vi "Hardware In - NI 9862 (NOx).vi"() -> ()   [LabVIEW 2015, in "ECS-RT.lvlib"]
uses:
  ECS-RT.lvlib
  Globals/NOx Global.vi
panel:
  out "NOx1 Data":T1={"NOx (ppm)"=0, "O2 (%)"=0.0, "Sensor Supply Status"=3, "Sensor Temperature Status"=12, "NOx Signal Status"=48, "O2 Signal Status"=192, "Heater Mode Status"=96, "Heater Circuit Status"=31, "NOx Circuit Status"=31, "O2 Circuit Status"=31, "NOx Sensor Module Present"=FALSE} {"Heater Mode Status" items=["AUTO MODE"=0, "HEATUP SLOPE 3 OR 4"=32, "HEATUP SLOPE 1 OR 2"=64, "HEATER OFF / PREHEAT"=96]; "O2 Circuit Status" items=["OPEN WIRE"=3, "SHORT CIRCUIT"=5, "NO ERROR"=31]; "NOx Circuit Status" items=["OPEN WIRE"=3, "SHORT CIRCUIT"=5, "NO ERROR"=31]; "Heater Circuit Status" items=["OPEN WIRE"=3, "SHORT CIRCUIT"=5, "NO ERROR"=31]; "Sensor Temperature Status" items=["NOT AT TEMPERATURE"=0, "AT TEMPERATURE"=4, "ERROR"=8, "NOT AVAILABLE"=12]; "O2 Signal Status" items=["NOT VALID"=0, "VALID"=64, "ERROR"=128, "NOT AVAILABLE"=192]; "NOx Signal Status" items=["NOT VALID"=0, "VALID"=16, "ERROR"=32, "NOT AVAILABLE"=48]; "Sensor Supply Status" items=["NOT IN RANGE", "SUPPLY IN RANGE", "ERROR", "NOT AVAILABLE"]}
  out "NOx2 Data":T1={"NOx (ppm)"=0, "O2 (%)"=0.0, "Sensor Supply Status"=3, "Sensor Temperature Status"=12, "NOx Signal Status"=48, "O2 Signal Status"=192, "Heater Mode Status"=96, "Heater Circuit Status"=31, "NOx Circuit Status"=31, "O2 Circuit Status"=31, "NOx Sensor Module Present"=FALSE} {"Heater Mode Status" items=["AUTO MODE"=0, "HEATUP SLOPE 3 OR 4"=32, "HEATUP SLOPE 1 OR 2"=64, "HEATER OFF / PREHEAT"=96]; "O2 Circuit Status" items=["OPEN WIRE"=3, "SHORT CIRCUIT"=5, "NO ERROR"=31]; "NOx Circuit Status" items=["OPEN WIRE"=3, "SHORT CIRCUIT"=5, "NO ERROR"=31]; "Heater Circuit Status" items=["OPEN WIRE"=3, "SHORT CIRCUIT"=5, "NO ERROR"=31]; "Sensor Temperature Status" items=["NOT AT TEMPERATURE"=0, "AT TEMPERATURE"=4, "ERROR"=8, "NOT AVAILABLE"=12]; "O2 Signal Status" items=["NOT VALID"=0, "VALID"=64, "ERROR"=128, "NOT AVAILABLE"=192]; "NOx Signal Status" items=["NOT VALID"=0, "VALID"=16, "ERROR"=32, "NOT AVAILABLE"=48]; "Sensor Supply Status" items=["NOT IN RANGE", "SUPPLY IN RANGE", "ERROR", "NOT AVAILABLE"]}
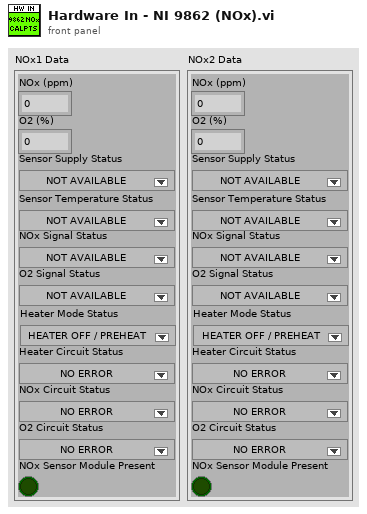
[diagram p1: front panel]
types:
  T1 = cluster{"NOx (ppm)":i16, "O2 (%)":sgl, "Sensor Supply Status":u8, "Sensor Temperature Status":u8, "NOx Signal Status":u8, "O2 Signal Status":u8, "Heater Mode Status":u8, "Heater Circuit Status":u8, "NOx Circuit Status":u8, "O2 Circuit Status":u8, "NOx Sensor Module Present":bool}
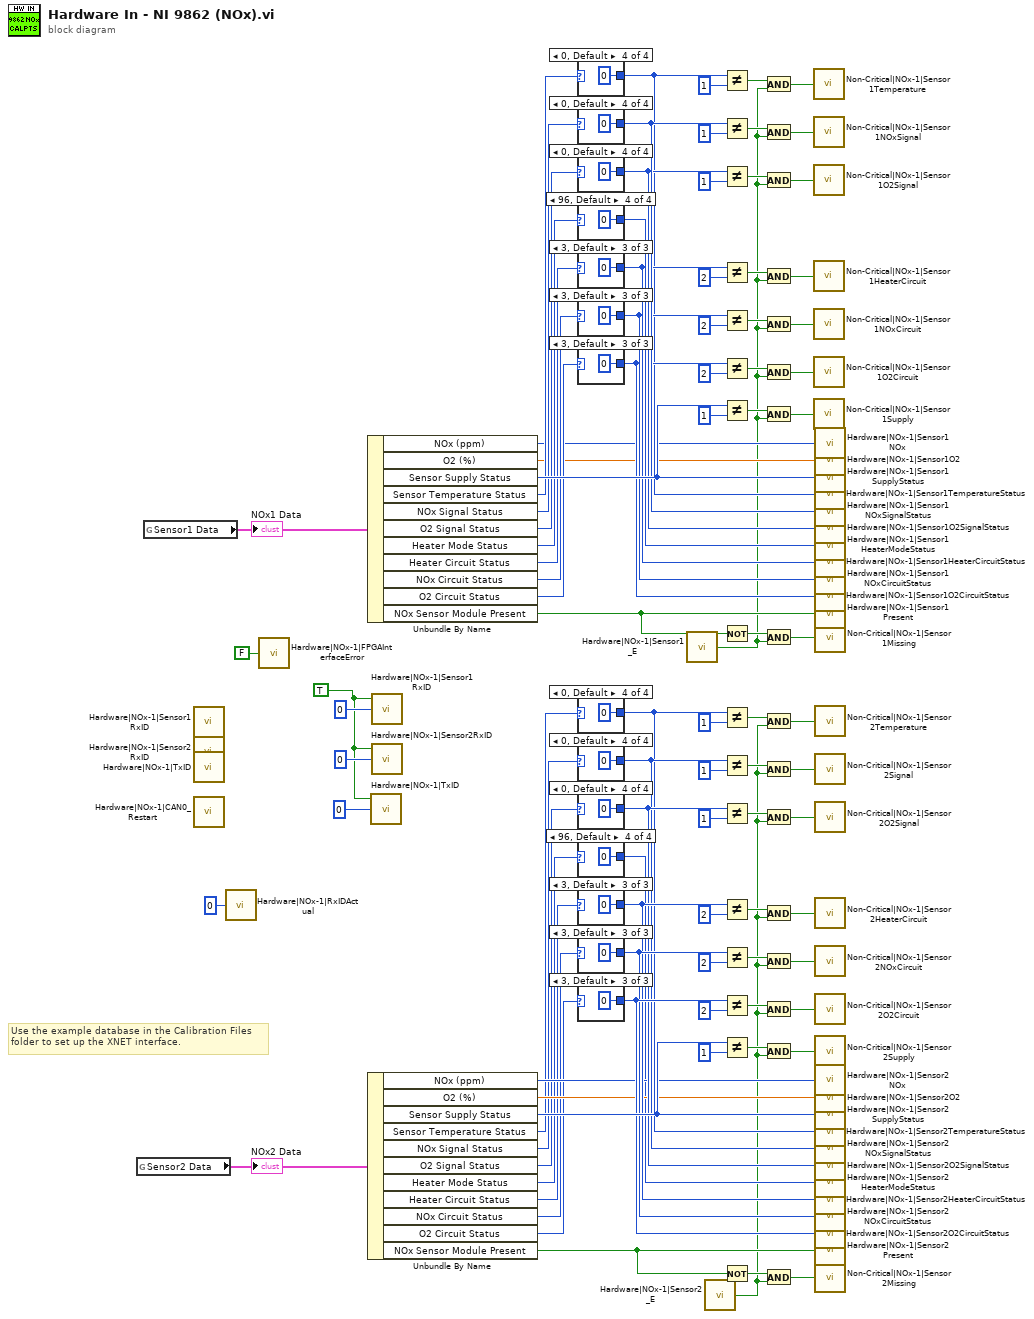
[diagram p0: block diagram]
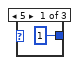
[diagram p2: hidden frame]
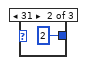
[diagram p3: hidden frame]
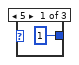
[diagram p4: hidden frame]
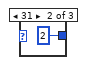
[diagram p5: hidden frame]
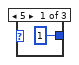
[diagram p6: hidden frame]
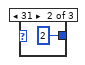
[diagram p7: hidden frame]
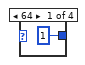
[diagram p8: hidden frame]
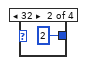
[diagram p9: hidden frame]
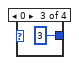
[diagram p10: hidden frame]
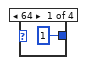
[diagram p11: hidden frame]
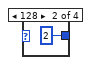
[diagram p12: hidden frame]
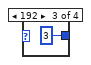
[diagram p13: hidden frame]
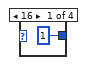
[diagram p14: hidden frame]
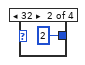
[diagram p15: hidden frame]
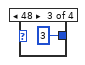
[diagram p16: hidden frame]
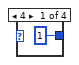
[diagram p17: hidden frame]
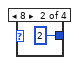
[diagram p18: hidden frame]
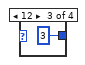
[diagram p19: hidden frame]
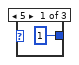
[diagram p20: hidden frame]
diagram:
  w3 = TRUE ("Adapt")
  # "Use the example database in the Calibration Files\nfolder to set up the XNET interface."
  n1 = global read "NOx Global.vi" "Sensor2 Data"() -> (w8:T1)
  "NOx2 Data" <- w8
  n2 = global read "NOx Global.vi" "Sensor1 Data"() -> (w7:T1)
  "NOx1 Data" <- w7
  n3 = call "Hardware|NOx-1|Sensor1RxID"() -> ()  [unwired: 1 out]
  n4 = call "Hardware|NOx-1|Sensor2RxID"() -> ()  [unwired: 1 out]
  n5 = call "Hardware|NOx-1|TxID"() -> ()  [unwired: 1 out]
  n6 = call "Hardware|NOx-1|CAN0_Restart"() -> ()  [unwired: 1 out]
  n7 = call "Hardware|NOx-1|RxIDActual"("Value"=u32 0) -> ()
  n8 = call "Hardware|NOx-1|FPGAInterfaceError"("Value"=FALSE) -> ()
  n9 = Unbundle By Name(w7) -> ("NOx (ppm)"=w43:i16, "O2 (%)"=w44:sgl, "Sensor Supply Status"=w76:u8, "Sensor Temperature Status"=w45:u8, "NOx Signal Status"=w46:u8, "O2 Signal Status"=w47:u8, "Heater Mode Status"=w48:u8, "Heater Circuit Status"=w49:u8, "NOx Circuit Status"=w50:u8, "O2 Circuit Status"=w51:u8, "NOx Sensor Module Present"=w77:bool)
  n10 = Unbundle By Name(w8) -> ("NOx (ppm)"=w61:i16, "O2 (%)"=w60:sgl, "Sensor Supply Status"=w91:u8, "Sensor Temperature Status"=w59:u8, "NOx Signal Status"=w58:u8, "O2 Signal Status"=w57:u8, "Heater Mode Status"=w55:u8, "Heater Circuit Status"=w54:u8, "NOx Circuit Status"=w53:u8, "O2 Circuit Status"=w52:u8, "NOx Sensor Module Present"=w92:bool)
  n11 = call "Hardware|NOx-1|TxID"("Value"=u32 0, "Adapt"=w3) -> ()  [unwired: 1 in]
  n12 = call "Hardware|NOx-1|Sensor1RxID"("Value"=u32 0, "Adapt"=w3) -> ()  [unwired: 1 in]
  n13 = call "Hardware|NOx-1|Sensor2RxID"("Value"=u32 0, "Adapt"=w3) -> ()  [unwired: 1 in]
  n14 = case shown="0, Default" w45 {
    tunnel: [1 2 3 0] -> w62
    frame 4 {
    }
    frame 8 {
    }
    frame 12 {
    }
    frame 0, Default {
    }
  }
  n15 = case shown="0, Default" w46 {
    tunnel: [1 2 3 0] -> w74
    frame 16 {
    }
    frame 32 {
    }
    frame 48 {
    }
    frame 0, Default {
    }
  }
  n16 = case shown="0, Default" w47 {
    tunnel: [1 2 3 0] -> w73
    frame 64 {
    }
    frame 128 {
    }
    frame 192 {
    }
    frame 0, Default {
    }
  }
  n17 = case shown="96, Default" w48 {
    tunnel: [1 2 3 0] -> w72
    frame 64 {
    }
    frame 32 {
    }
    frame 0 {
    }
    frame 96, Default {
    }
  }
  n18 = case shown="3, Default" w49 {
    tunnel: [1 2 0] -> w71
    frame 5 {
    }
    frame 31 {
    }
    frame 3, Default {
    }
  }
  n19 = case shown="3, Default" w50 {
    tunnel: [1 2 0] -> w70
    frame 5 {
    }
    frame 31 {
    }
    frame 3, Default {
    }
  }
  n20 = case shown="3, Default" w51 {
    tunnel: [1 2 0] -> w69
    frame 5 {
    }
    frame 31 {
    }
    frame 3, Default {
    }
  }
  n21 = case shown="0, Default" w59 {
    tunnel: [1 2 3 0] -> w85
    frame 4 {
    }
    frame 8 {
    }
    frame 12 {
    }
    frame 0, Default {
    }
  }
  n22 = case shown="0, Default" w58 {
    tunnel: [1 2 3 0] -> w86
    frame 16 {
    }
    frame 32 {
    }
    frame 48 {
    }
    frame 0, Default {
    }
  }
  n23 = case shown="0, Default" w57 {
    tunnel: [1 2 3 0] -> w87
    frame 64 {
    }
    frame 128 {
    }
    frame 192 {
    }
    frame 0, Default {
    }
  }
  n24 = case shown="96, Default" w55 {
    tunnel: [1 2 3 0] -> w56
    frame 64 {
    }
    frame 32 {
    }
    frame 0 {
    }
    frame 96, Default {
    }
  }
  n25 = case shown="3, Default" w54 {
    tunnel: [1 2 0] -> w88
    frame 5 {
    }
    frame 31 {
    }
    frame 3, Default {
    }
  }
  n26 = case shown="3, Default" w53 {
    tunnel: [1 2 0] -> w89
    frame 5 {
    }
    frame 31 {
    }
    frame 3, Default {
    }
  }
  n27 = case shown="3, Default" w52 {
    tunnel: [1 2 0] -> w90
    frame 5 {
    }
    frame 31 {
    }
    frame 3, Default {
    }
  }
  n28 = call "Hardware|NOx-1|Sensor1_E"() -> ("Value"=w9:bool)
  n29 = call "Hardware|NOx-1|Sensor2_E"() -> ("Value"=w26:bool)
  n30 = Not Equal?(x=w62, y=1) -> (x != y?=w24:bool)
  n31 = Not Equal?(x=w74, y=1) -> (x != y?=w15:bool)
  n32 = Not Equal?(x=w73, y=1) -> (x != y?=w14:bool)
  n33 = Not Equal?(x=w71, y=2) -> (x != y?=w13:bool)
  n34 = Not Equal?(x=w70, y=2) -> (x != y?=w12:bool)
  n35 = Not Equal?(x=w69, y=2) -> (x != y?=w11:bool)
  n36 = Not Equal?(x=w76, y=1) -> (x != y?=w10:bool)
  n37 = Not(x=w77) -> (.not. x?=w22:bool)
  n38 = Not Equal?(x=w85, y=1) -> (x != y?=w34:bool)
  n39 = Not Equal?(x=w86, y=1) -> (x != y?=w33:bool)
  n40 = Not Equal?(x=w87, y=1) -> (x != y?=w32:bool)
  n41 = Not Equal?(x=w88, y=2) -> (x != y?=w31:bool)
  n42 = Not Equal?(x=w89, y=2) -> (x != y?=w30:bool)
  n43 = Not Equal?(x=w90, y=2) -> (x != y?=w29:bool)
  n44 = Not Equal?(x=w91, y=1) -> (x != y?=w28:bool)
  n45 = Not(x=w92) -> (.not. x?=w27:bool)
  n46 = And(x=w24, y=w9) -> (x .and. y?=w25:bool)
  n47 = And(x=w15, y=w9) -> (x .and. y?=w16:bool)
  n48 = And(x=w14, y=w9) -> (x .and. y?=w17:bool)
  n49 = And(x=w13, y=w9) -> (x .and. y?=w18:bool)
  n50 = And(x=w12, y=w9) -> (x .and. y?=w19:bool)
  n51 = And(x=w11, y=w9) -> (x .and. y?=w21:bool)
  n52 = And(x=w10, y=w9) -> (x .and. y?=w20:bool)
  n53 = And(x=w22, y=w9) -> (x .and. y?=w23:bool)
  n54 = And(x=w34, y=w26) -> (x .and. y?=w42:bool)
  n55 = And(x=w33, y=w26) -> (x .and. y?=w41:bool)
  n56 = And(x=w32, y=w26) -> (x .and. y?=w40:bool)
  n57 = And(x=w31, y=w26) -> (x .and. y?=w39:bool)
  n58 = And(x=w30, y=w26) -> (x .and. y?=w38:bool)
  n59 = And(x=w29, y=w26) -> (x .and. y?=w37:bool)
  n60 = And(x=w28, y=w26) -> (x .and. y?=w36:bool)
  n61 = And(x=w27, y=w26) -> (x .and. y?=w35:bool)
  n62 = call "Non-Critical|NOx-1|Sensor1Temperature"("Fault"=w25) -> ()  [unwired: 2 in]
  n63 = call "Non-Critical|NOx-1|Sensor1NOxSignal"("Fault"=w16) -> ()  [unwired: 2 in]
  n64 = call "Non-Critical|NOx-1|Sensor1O2Signal"("Fault"=w17) -> ()  [unwired: 2 in]
  n65 = call "Non-Critical|NOx-1|Sensor1HeaterCircuit"("Fault"=w18) -> ()  [unwired: 2 in]
  n66 = call "Non-Critical|NOx-1|Sensor1NOxCircuit"("Fault"=w19) -> ()  [unwired: 2 in]
  n67 = call "Non-Critical|NOx-1|Sensor1O2Circuit"("Fault"=w21) -> ()  [unwired: 2 in]
  n68 = call "Non-Critical|NOx-1|Sensor1Supply"("Fault"=w20) -> ()  [unwired: 2 in]
  n69 = call "Hardware|NOx-1|Sensor1NOx"("Value"=w43) -> ()
  n70 = call "Hardware|NOx-1|Sensor1O2"("Value"=w44) -> ()
  n71 = call "Hardware|NOx-1|Sensor1SupplyStatus"("Value"=w76) -> ()
  n72 = call "Hardware|NOx-1|Sensor1TemperatureStatus"("Value"=w62) -> ()
  n73 = call "Hardware|NOx-1|Sensor1NOxSignalStatus"("Value"=w74) -> ()
  n74 = call "Hardware|NOx-1|Sensor1O2SignalStatus"("Value"=w73) -> ()
  n75 = call "Hardware|NOx-1|Sensor1HeaterModeStatus"("Value"=w72) -> ()
  n76 = call "Hardware|NOx-1|Sensor1HeaterCircuitStatus"("Value"=w71) -> ()
  n77 = call "Hardware|NOx-1|Sensor1NOxCircuitStatus"("Value"=w70) -> ()
  n78 = call "Hardware|NOx-1|Sensor1O2CircuitStatus"("Value"=w69) -> ()
  n79 = call "Hardware|NOx-1|Sensor1Present"("Value"=w77) -> ()
  n80 = call "Non-Critical|NOx-1|Sensor1Missing"("Fault"=w23) -> ()  [unwired: 2 in]
  n81 = call "Non-Critical|NOx-1|Sensor2Temperature"("Fault"=w42) -> ()  [unwired: 2 in]
  n82 = call "Non-Critical|NOx-1|Sensor2Signal"("Fault"=w41) -> ()  [unwired: 2 in]
  n83 = call "Non-Critical|NOx-1|Sensor2O2Signal"("Fault"=w40) -> ()  [unwired: 2 in]
  n84 = call "Non-Critical|NOx-1|Sensor2HeaterCircuit"("Fault"=w39) -> ()  [unwired: 2 in]
  n85 = call "Non-Critical|NOx-1|Sensor2NOxCircuit"("Fault"=w38) -> ()  [unwired: 2 in]
  n86 = call "Non-Critical|NOx-1|Sensor2O2Circuit"("Fault"=w37) -> ()  [unwired: 2 in]
  n87 = call "Non-Critical|NOx-1|Sensor2Supply"("Fault"=w36) -> ()  [unwired: 2 in]
  n88 = call "Hardware|NOx-1|Sensor2NOx"("Value"=w61) -> ()
  n89 = call "Hardware|NOx-1|Sensor2O2"("Value"=w60) -> ()
  n90 = call "Hardware|NOx-1|Sensor2SupplyStatus"("Value"=w91) -> ()
  n91 = call "Hardware|NOx-1|Sensor2TemperatureStatus"("Value"=w85) -> ()
  n92 = call "Hardware|NOx-1|Sensor2NOxSignalStatus"("Value"=w86) -> ()
  n93 = call "Hardware|NOx-1|Sensor2O2SignalStatus"("Value"=w87) -> ()
  n94 = call "Hardware|NOx-1|Sensor2HeaterModeStatus"("Value"=w56) -> ()
  n95 = call "Hardware|NOx-1|Sensor2HeaterCircuitStatus"("Value"=w88) -> ()
  n96 = call "Hardware|NOx-1|Sensor2NOxCircuitStatus"("Value"=w89) -> ()
  n97 = call "Hardware|NOx-1|Sensor2O2CircuitStatus"("Value"=w90) -> ()
  n98 = call "Hardware|NOx-1|Sensor2Present"("Value"=w92) -> ()
  n99 = call "Non-Critical|NOx-1|Sensor2Missing"("Fault"=w35) -> ()  [unwired: 2 in]
